vi "Layout Popup.vi"(6 "Height (200)":i16=200, 7 "Initial? (F)":bool, 8 "error in (no error)":errorcluster, 10 "Popup VI In":refnum<vi>, 11 "String Control In":refnum<vi>) -> (0 "error out":errorcluster, 2 "Popup VI":refnum<vi>, 3 "String Control":refnum<vi>)   [LabVIEW 2020, in "AutoComplete.lvlib"]
uses:
  AutoComplete.lvlib
  <vilib>/Utility/miscctls.llb/LVRectTypeDef.ctl
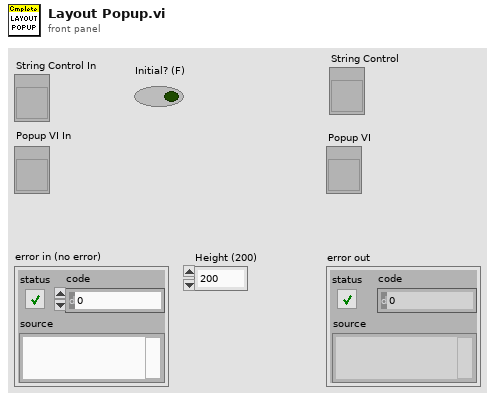
[diagram p1: front panel]
types:
  T1 = typedef "LVRectTypeDef.ctl" = cluster{"Left":i16, "Top":i16, "Right":i16, "Bottom":i16}
  T2 = enum32{"Invalid", "Standard", "Closed", "Hidden", "Minimized", "Maximized"}
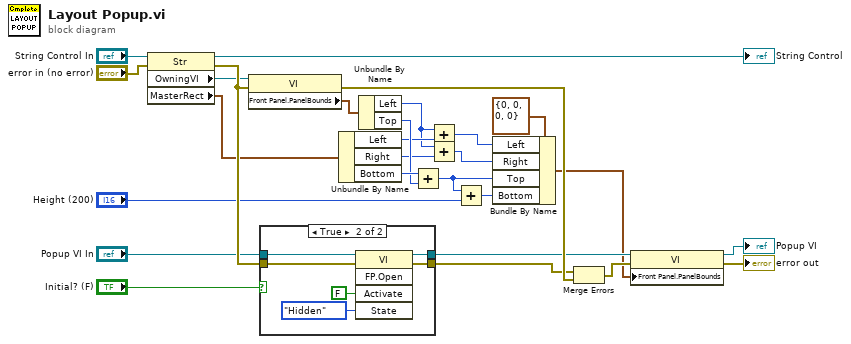
[diagram p0: block diagram]
diagram:
  n1 = property class="Str"(reference="String Control In", error in="error in (no error)") -> (reference out=→"String Control":refnum<vi>, error out=w25:errorcluster, "OwningVI"=w22:refnum<vi>, "MasterRect"=w21:T1)
  n2 = property class="VI"(reference=w22, error in=w25) -> (error out=w27:errorcluster, "Front Panel.PanelBounds"=w20:T1)  [unwired: 1 out]
  n3 = case shown="True" "Initial? (F)" {
    tunnel: w25 -> [w28 w35]
    tunnel: [w29 w33] -> w24
    tunnel: "Popup VI In" -> [w29 w31]
    tunnel: [w28 w30] -> w2
    frame False {
    }
    frame True {
      n4 = invoke class="VI" method="FP.Open"(reference=w31, error in=w35, "Activate"=FALSE ("Activate?"), "State"=T2."Hidden") -> (reference out=w33:refnum<vi>, error out=w30:errorcluster)  [unwired: 1 in, 3 out]
    }
  }
  n5 = Unbundle By Name(w21) -> ("Left"=w15:i16, "Right"=w16:i16, "Bottom"=w19:i16)
  n6 = Unbundle By Name(w20) -> ("Left"=w14:i16, "Top"=w17:i16)
  n7 = Add(x=w19, y=w17) -> (x+y=w18:i16)
  n8 = Add(x=w14, y=w15) -> (x+y=w10:i16)
  n9 = Add(x=w14, y=w16) -> (x+y=w11:i16)
  n10 = Add(x=w18, y="Height (200)") -> (x+y=w23:i16)
  n11 = Bundle By Name(cluster=T1 {"Left"=0, "Top"=0, "Right"=0, "Bottom"=0} ("Front Panel Window:Panel Bounds"), "Left"=w10, "Right"=w11, "Top"=w18, "Bottom"=w23) -> (w13:T1)
  n12 = Merge Errors(w2, w27) -> (w26:errorcluster)
  n13 = property class="VI"(reference=w24, error in=w26, "Front Panel.PanelBounds"=w13) -> (reference out=→"Popup VI":refnum<vi>, error out=→"error out":errorcluster)
